vi "Transition Measurements N chan (obs).vi"(6 "percent level settings":T3={"method"=enum."auto select", "histogram size"=256, "histogram method"=enum."mode", "reserved"=1.0} {"reserved" format="%0.2f"}, 7 "edge number (1)":i32=1 min=1, 8 "error in (no error)":errorcluster, 9 "reference levels":T2={"high ref level"=90.0, "mid ref level"=50.0, "low ref level"=10.0, "ref units"=1} {"ref units" items=["absolute", "percent"]; "high ref level" format="%.2p"; "low ref level" format="%.2p"; "mid ref level" format="%.2p"}, 10 "polarity (rising)":u16(ring)=1 items=["falling", "rising"], 11 "signal(s) in":waveform(dbl)[](array[waveform])) -> (0 "error out":errorcluster, 1 "overshoot (%)":dbl[](array[numeric]) format="%.2p", 2 "preshoot (%)":dbl[](array[numeric]) format="%.2p", 3 "duration":dbl[](array[numeric]) format="%.2p", 4 "measurement info":T1(array[cluster]), 5 "slew rate":dbl[](array[numeric]) format="%.2p")   [LabVIEW 2020, in "NI_MAPro.lvlib"]
uses:
  NI_MAPro.lvlib
  NI_MABase.lvlib
panel:
  # "This VI is obsolete !!!\nYou should replace this VI in your diagram with the Transition Measurement 1 chan VI.  \n\nNOTE: If you have wired to the output of this obsolete VI, \n           please be aware that the new Transition Measurement 1 chan VI:\n           1. Use two new clusters, pre-transition and under-transtion, to replace preshoot(%) and overshoot(%).\n           2. Change the output name slew rate to slope.\n           3. Change the output name duration to transition duration."
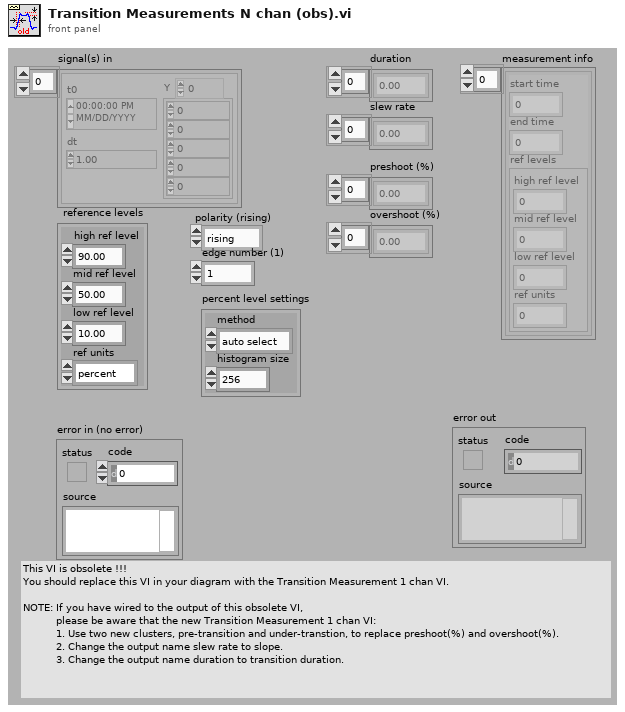
[diagram p1: front panel]
types:
  T1 = cluster{"start time":dbl, "end time":dbl, "ref levels":cluster{"high ref level":dbl, "mid ref level":dbl, "low ref level":dbl, "ref units":u16}}[]
  T2 = cluster{"high ref level":dbl, "mid ref level":dbl, "low ref level":dbl, "ref units":u16}
  T3 = cluster{"method":enum32{"histogram", "peak", "auto select"}, "histogram size":i32, "histogram method":enum16{"mode"}, "reserved":dbl}
  T4 = cluster{"start time":dbl, "end time":dbl, "ref levels":cluster{"high ref level":dbl, "mid ref level":dbl, "low ref level":dbl, "ref units":u16}}
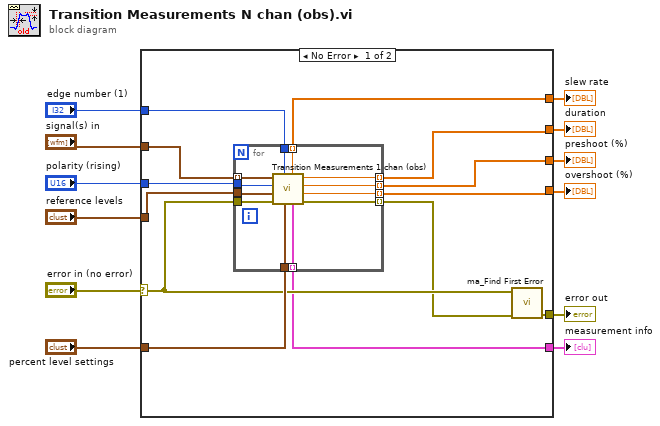
[diagram p0: block diagram]
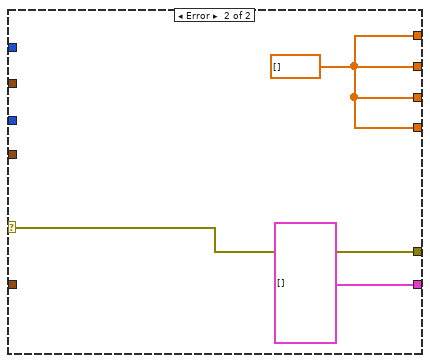
[diagram p2: hidden frame]
diagram:
  n1 = case shown="No Error" "error in (no error)" {
    selector: "error in (no error)" -> [w19 w40]
    tunnel: "percent level settings" -> [w24 _]
    tunnel: [w23 w40] -> w10
    tunnel: "signal(s) in" -> [w25 _]
    tunnel: [w17 w38] -> w8
    tunnel: "reference levels" -> [w22 _]
    tunnel: "edge number (1)" -> [w21 _]
    tunnel: "polarity (rising)" -> [w20 _]
    tunnel: [w18 w38] -> w4
    tunnel: [w13 T1 []] -> w3
    tunnel: [w16 w38] -> w2
    tunnel: [w15 w38] -> w1
    frame No Error {
      n2 = for {
        tunnel: w19 -> [w33]
        tunnel: w24 -> [w27]
        tunnel: w25 -> [w36] mode=indexing
        tunnel: w22 -> [w34]
        tunnel: w21 -> [w37]
        tunnel: w20 -> [w35]
        tunnel: [w32] -> w18 mode=indexing
        tunnel: [w31] -> w17 mode=indexing
        tunnel: [w30] -> w16 mode=indexing
        tunnel: [w29] -> w15 mode=indexing
        tunnel: [w28] -> w14 mode=indexing
        tunnel: [w26] -> w13 mode=indexing
        n3 = call "Transition Measurements 1 chan (obs).vi"("percent level settings"=w27, "edge number (1)"=w37, "error in (no error)"=w33, "reference levels"=w34, "polarity (rising)"=w35, "signal in"=w36) -> ("error out"=w28:errorcluster, "overshoot (%)"=w29:dbl, "preshoot (%)"=w30:dbl, "duration"=w31:dbl, "measurement info"=w26:T4, "slew rate"=w32:dbl)
      }
      n4 = call "ma_Find First Error.vi"("error array in"=w14, "error in 1 (no error)"=w19) -> ("error out"=w23:errorcluster)  [unwired: 2 in, 3 out]
    }
    frame Error {
      w38 = dbl[] []
    }
  }
  "error out" <- w10
  "duration" <- w8
  "slew rate" <- w4
  "measurement info" <- w3
  "overshoot (%)" <- w1
  "preshoot (%)" <- w2
